vi "VisBx Anzeige PNS.vi"() -> ()   [LabVIEW 2020, in "PNS.lvlib" / "PNS Anlagenuebersicht.lvlib"]
uses:
  PNS Anlagenuebersicht.lvlib
  Visualisierungs Elemente/Zahlen-Ausgabefeld.ctl
  Aktionen FGV Loopkennung.ctl
  Aktionen FGV Grenzwerte.ctl
  Seiten/System Einstellungen V2/Aktioen FGV System.ctl
  PNS Ausgabefelder einfaerben Aktionen.ctl
  <vilib>/Utility/miscctls.llb/LVPointTypeDef.ctl
  Stoerungen/FGV Stoerung aufnehmen Aktion.ctl
  Aktionen FGV Istwerte.ctl
  <vilib>/picture/picture.llb/Draw True-Color Pixmap.vi
  PNS.lvlib
  Allgemein/allgemeine Sub-VIs.lvlib
  Seiten/Anlagenuebersicht/VisBx Anzeige/TDMS laden/TDMS laden.lvlib
  Seiten/Anlagenuebersicht/VisBx Anzeige/VisBx Anzeige.lvlib
  Stoerungen/Stoerungen.lvlib
  Seiten/System Einstellungen V2/System Einstellungen V2.lvlib
  Seiten/Anlagenuebersicht/VisBx Anzeige/Anlagenuebersicht.lvlib
panel:
  out "maxLoop":i32=10
  out "PNS Inaktiv":string
  out "Komm":string
  out "Druckluft":string
  in  "Fehler":string="Die Umgebungsvariable besitzt\nnicht den selben Datentyp wie\ndie TDMS-Datei."
  out "°C":T1
  out "°C":T1
  out "°C":T1
  out "°C":T1
  out "°C":T1
  out "°C":T1
  out "°C":T1
  out "°C":T1
  out "Bild":picture
  # "Anlagenübersicht PNS"
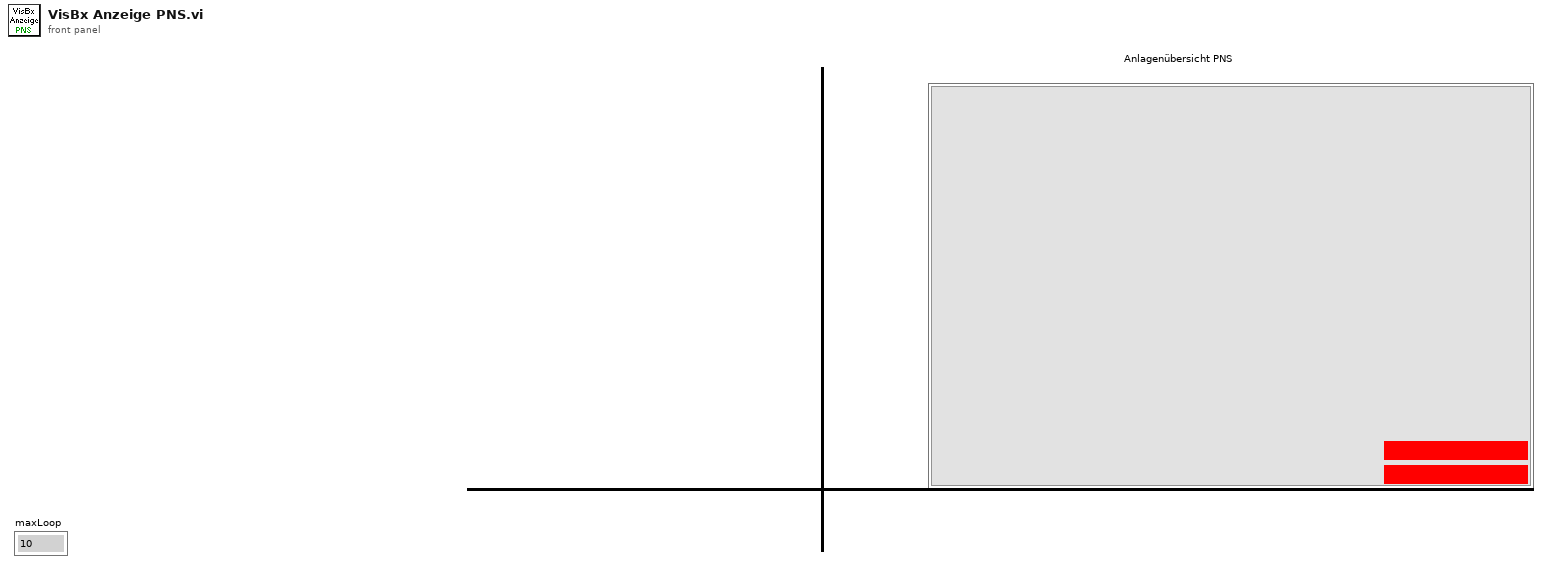
[diagram p1: front panel]
types:
  T1 = typedef "Zahlen-Ausgabefeld.ctl" = sgl
  T2 = typedef "PNS.lvlib/Aktionen FGV Loopkennung.ctl" = enum16{"lesen", "schreiben"}
  T3 = typedef "PNS.lvlib/PNS Anlagenuebersicht.lvlib/PNS Ausgabefelder einfaerben Aktionen.ctl" = enum16{"lesen", "prüfen", "initialisieren"}
  T4 = typedef "System Einstellungen V2.lvlib/Aktioen FGV System.ctl" = enum16{"lesen", "laden", "speichern", "Optionen schreiben", "Zeitstempel", "Reset BMP", "Reset SQP", "Wartung", "Werkseinstellung"}
  T5 = typedef "PNS.lvlib/Aktionen FGV Grenzwerte.ctl" = enum16{"lesen", "Grenzw. schreiben", "Anweisungscode", "IP-Adresse", "laden", "speichern", "Anweisungscode vorgeben"}
  T6 = typedef "LVPointTypeDef.ctl" = cluster{"Horizontal":i16, "Vertical":i16}
  T7 = typedef "PNS.lvlib/PNS Geraetekennung.ctl" = cluster{"Loops":string[], "Gerätetype":string, "Loopkennung":u16[], "Seriennummer":string, "Geraetekennung":u16, "SoftWare Version":string, "LP Kennung":u16}
  T8 = typedef "System Einstellungen V2.lvlib/Optionen.ctl" = cluster{"Störmeldep.":bool, "Betriebszustände":bool, "LN2 Befüllung":bool, "Klimaanlage ?":bool, "AK in ppm":bool, "log Cal-Gas":bool, "log 0-Gas":bool, "log CG zu PNS":bool, "Reserve":bool, "Durchflusssensor 0-5V":bool, "PNS?":bool, "Container":bool, "Mit N2 spülen":bool, "Span Gas Auswahl":T9, "VFS 1":bool, "VFS 2":bool, "VFS 3":bool, "VFS 4":bool, "TRE08":bool, "Leakcheck vor Kal":bool, "Amium 10-Fach":bool, "Verticale Scrollbar aktiv":bool, "Loggingtakt":bool, "SP laden speichern":u16}
  T9 = typedef "Funktionstasten.lvlib/Spaneingang.ctl" = u16
  T10 = typedef "Steuerung PNS.lvclass/Anlegengrenzwerte PNS.ctl" = cluster{"Filter:":T11, "Ventilplatte:":T11, "Heizleitung 1:":T11, "Heizleitung 2:":T11, "Heizleitung 3:":T11, "Heizleitung 4:":T11, "Heizleitung 5:":T11, "Heizleitung 6:":T11}
  T11 = typedef "Steuerung PNS.lvclass/Anlagengrenzwerte Parameteranzeige.ctl" = cluster{"Sollwert":T12, "Warn-Min":T12, "Warn-Max":T12, "Abschalt-Min":T12, "Abschalt-Max":T12, "Regler":u16, "AnlagenParameter":string}
  T12 = typedef "Zahlen-Eingabefeld.ctl" = sgl
  T13 = typedef "VisParam-Typdef.lvlib/VisSchritt.ctl" = cluster{"Schritt-Typ":T14, "Schritt-Daten":variant}
  T14 = typedef "VisParam-Typdef.lvlib/VisSchritt-Typ.ctl" = enum16{"leer", "Punkt", "Linie", "Linienzug", "Fixtext", "Textrechteck", "Ziffernanzeige", "Rechteck", "Rechteck rund", "Ellipse", "Bogen", "Kreis", "Pixmap"}
  T15 = typedef "Anlagenuebersicht.lvlib/VisBx Anzeige.lvlib/TDMS laden.lvlib/TDMS-Eigenschaften.ctl" = cluster{"Größe":T16, "URL":string, "Raster":i16, "Hintergrund":u32}
  T16 = typedef "LVBoundsTypeDef.ctl" = cluster{"Width":u32, "Height":u32}
  T17 = typedef "PNS.lvlib/Aktionen FGV Istwerte.ctl" = enum16{"lesen", "initialisieren", "schreiben", "Störungen"}
  T18 = typedef "Stoerungen.lvlib/FGV Stoerung aufnehmen Aktion.ctl" = enum16{"Initialisieren", "Schreiben", "Lesen", "Quittieren", "quit. löschen"}
  T19 = typedef "Steuerung PNS.lvclass/Regler.ctl" = cluster{"Istwert":i16, "Sollwert":i16, "Alarm MIN":i16, "Alarm MAX":i16, "Regler sperren":i16, "Analog Ausgang":i16}[]
  T20 = cluster{"Istwert":i16, "Sollwert":i16, "Alarm MIN":i16, "Alarm MAX":i16, "Regler sperren":i16, "Analog Ausgang":i16}
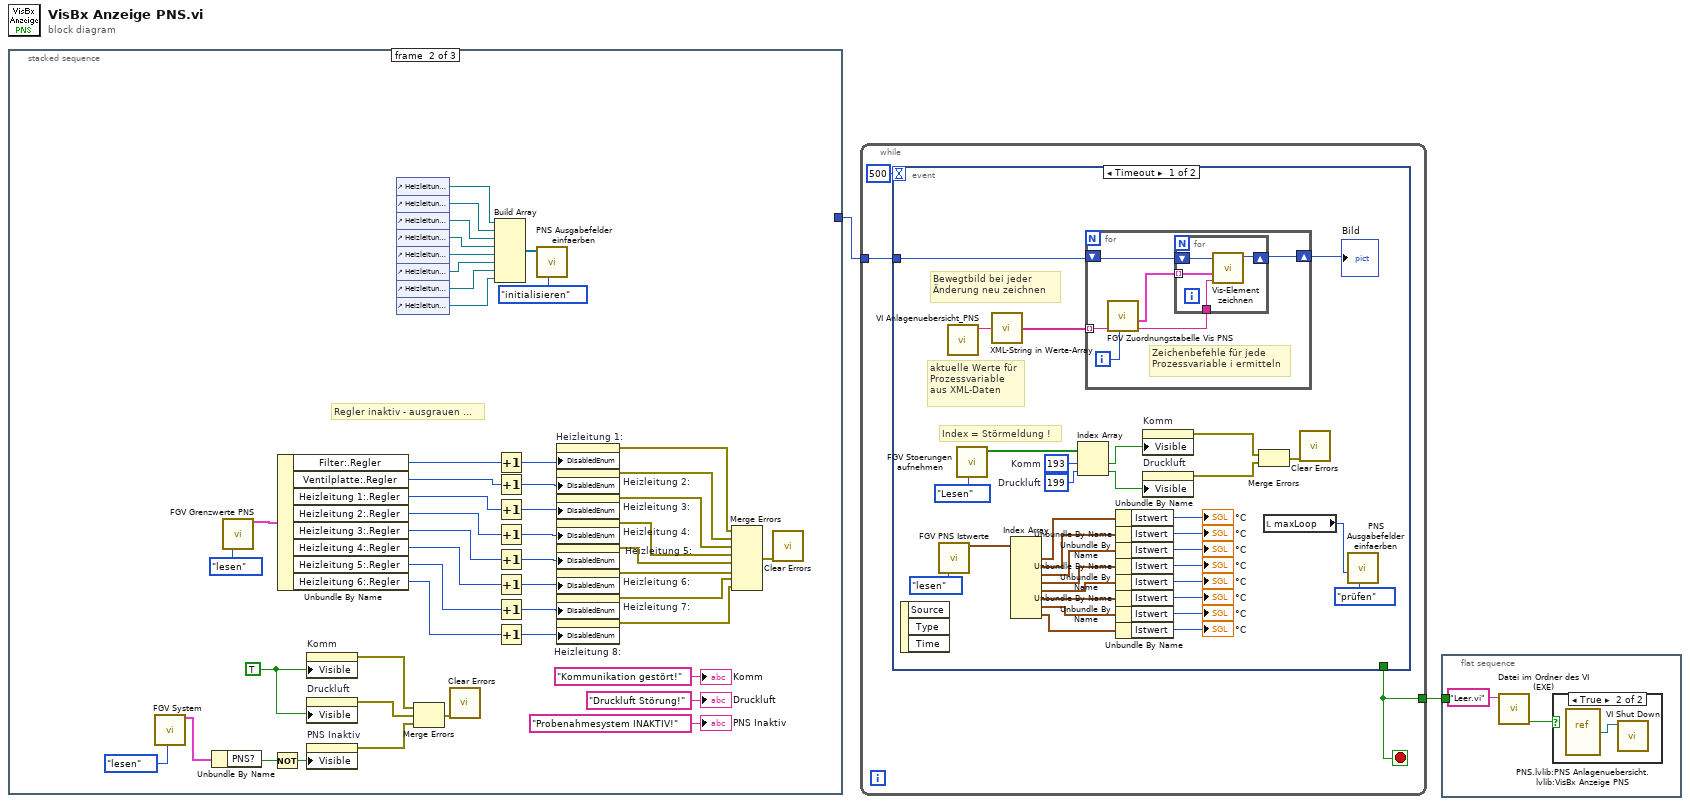
[diagram p0: block diagram]
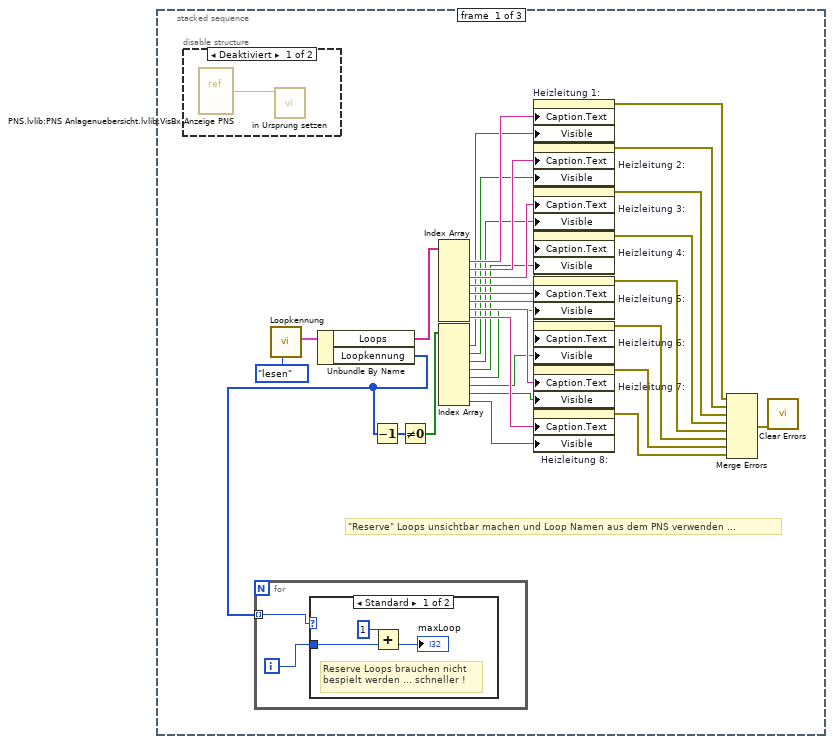
[diagram p3: hidden frame]
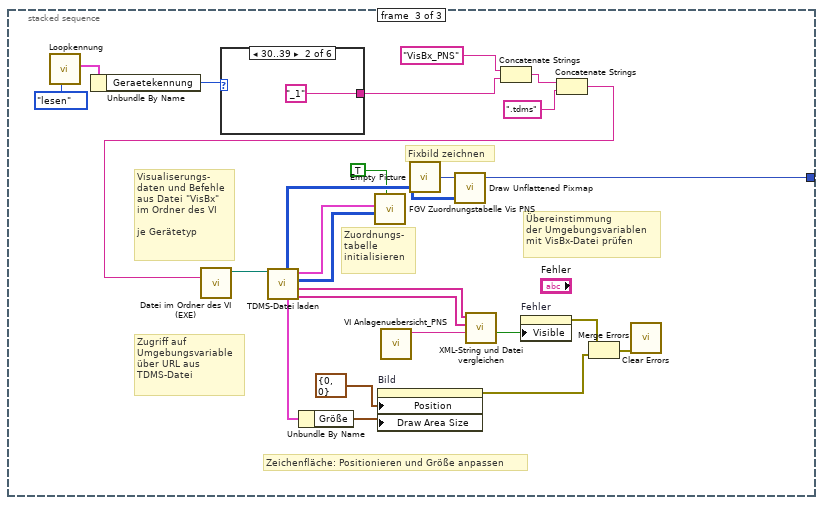
[diagram p6: hidden frame]
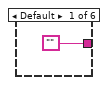
[diagram p7: hidden frame]
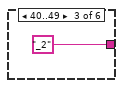
[diagram p8: hidden frame]
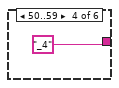
[diagram p9: hidden frame]
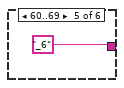
[diagram p10: hidden frame]
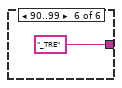
[diagram p11: hidden frame]
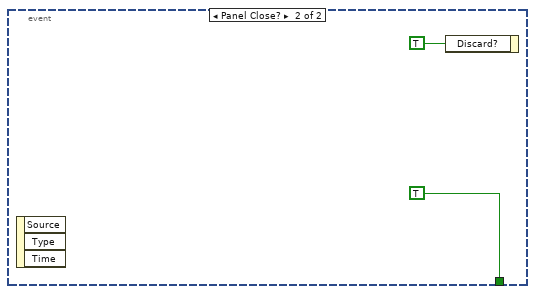
[diagram p12: hidden frame]
diagram:
  n1 = stacked-sequence {
    tunnel: [_ _ w105] -> w2
    frame #0 {
      # "\"Reserve\" Loops unsichtbar machen und Loop Namen aus dem PNS verwenden ..."
      n2 = disable-structure shown="Deaktiviert" {
        frame Disabled {
          n3 = vi-ref "PNS.lvlib:PNS Anlagenuebersicht.lvlib:VisBx Anzeige PNS.vi"() -> (w39:refnum<vi>)
          n4 = call "in Ursprung setzen.vi"("VI Referenz"=w39) -> ()  [unwired: 11 in]
        }
        frame Enabled {
        }
      }
      n5 = call "Loopkennung.vi"("Aktion"=Aktionen_FGV_Loopkennung."lesen") -> ("LoopGeraetekennung"=w32:T7)  [unwired: 9 in, 1 out]
      n6 = Unbundle By Name(w32) -> ("Loops"=w31:string[], "Loopkennung"=w3:u16[])
      n7 = for {
        tunnel: w3 -> [w35] mode=indexing
        i -> [w34]
        n8 = case shown="Standard" w35 {
          tunnel: w34 -> [w38 _]
          frame Default {
            # "Reserve Loops brauchen nicht\nbespielt werden ... schneller !"
            n9 = Add(x=1, y=w38) -> (x+y=→"maxLoop":i32)
          }
          frame 1 {
            # "Reserve Loop,\nmaxLoop nicht mehr \nhoch zählen ..."
          }
        }
      }
      n10 = Decrement(x=w3) -> (x-1=w13:u16[])
      n11 = Not Equal To 0?(x=w13) -> (x != 0?=w12:bool[])
      n12 = Index Array(array=w31) -> (element #1=w23:string, element #2=w24:string, element #3=w25:string, element #4=w26:string, element #5=w30:string, element #6=w29:string, element #7=w28:string, element #8=w27:string)  [unwired: 8 in]
      n13 = Index Array(array=w12) -> (element #1=w11:bool, element #2=w10:bool, element #3=w9:bool, element #4=w8:bool, element #5=w7:bool, element #6=w6:bool, element #7=w5:bool, element #8=w4:bool)  [unwired: 8 in]
      n14 = property on="Heizleitung 1:" class="DigWert (strikt)"("Caption.Text"=w23, "Visible"=w11) -> (error out=w21:errorcluster)  [unwired: 2 in, 1 out]
      n15 = property on="Heizleitung 2:" class="DigWert (strikt)"("Caption.Text"=w24, "Visible"=w10) -> (error out=w20:errorcluster)  [unwired: 2 in, 1 out]
      n16 = property on="Heizleitung 3:" class="DigWert (strikt)"("Caption.Text"=w25, "Visible"=w9) -> (error out=w19:errorcluster)  [unwired: 2 in, 1 out]
      n17 = property on="Heizleitung 4:" class="DigWert (strikt)"("Caption.Text"=w26, "Visible"=w8) -> (error out=w18:errorcluster)  [unwired: 2 in, 1 out]
      n18 = property on="Heizleitung 5:" class="DigWert (strikt)"("Caption.Text"=w30, "Visible"=w7) -> (error out=w17:errorcluster)  [unwired: 2 in, 1 out]
      n19 = property on="Heizleitung 6:" class="DigWert (strikt)"("Caption.Text"=w29, "Visible"=w6) -> (error out=w16:errorcluster)  [unwired: 2 in, 1 out]
      n20 = property on="Heizleitung 7:" class="DigWert (strikt)"("Caption.Text"=w28, "Visible"=w5) -> (error out=w15:errorcluster)  [unwired: 2 in, 1 out]
      n21 = property on="Heizleitung 8:" class="DigWert (strikt)"("Caption.Text"=w27, "Visible"=w4) -> (error out=w14:errorcluster)  [unwired: 2 in, 1 out]
      n22 = Merge Errors(w21, w20, w19, w18, w17, w16, w15, w14) -> (w22:errorcluster)
      n23 = call <vilib>:"Clear Errors.vi"("error in (no error)"=w22) -> ()  [unwired: 5 in, 2 out]
    }
    frame #1 {
      w54 = TRUE
      # "Regler inaktiv - ausgrauen ..."
      n24 = call "FGV System.vi"("Aktionen"=Aktioen_FGV_System."lesen") -> ("Optionen"=w53:T8)  [unwired: 12 in, 6 out]
      n25 = Unbundle By Name(w53) -> ("PNS?"=w51:bool)
      n26 = call "FGV Grenzwerte PNS.vi"("Aktionen FGV Grenzwerte"=Aktionen_FGV_Grenzwerte."lesen") -> ("Grenzwerte PNS 2"=w79:T10)  [unwired: 12 in, 2 out]
      n27 = Not(x=w51) -> (.not. x?=w68:bool)
      n28 = Unbundle By Name(w79) -> ("Filter:.Regler"=w78:u16, "Ventilplatte:.Regler"=w77:u16, "Heizleitung 1:.Regler"=w76:u16, "Heizleitung 2:.Regler"=w75:u16, "Heizleitung 3:.Regler"=w74:u16, "Heizleitung 4:.Regler"=w73:u16, "Heizleitung 5:.Regler"=w72:u16, "Heizleitung 6:.Regler"=w81:u16)
      n29 = property on="Komm" class="Str"("Visible"=w54) -> (error out=w66:errorcluster)  [unwired: 2 in, 1 out]
      n30 = property on="Druckluft" class="Str"("Visible"=w54) -> (error out=w65:errorcluster)  [unwired: 2 in, 1 out]
      n31 = property on="PNS Inaktiv" class="Str"("Visible"=w68) -> (error out=w64:errorcluster)  [unwired: 2 in, 1 out]
      n32 = control-ref of="Heizleitung 1:"() -> (w46:refnum<vi>)
      n33 = control-ref of="Heizleitung 2:"() -> (w48:refnum<vi>)
      n34 = control-ref of="Heizleitung 3:"() -> (w47:refnum<vi>)
      n35 = control-ref of="Heizleitung 4:"() -> (w44:refnum<vi>)
      n36 = control-ref of="Heizleitung 5:"() -> (w43:refnum<vi>)
      n37 = control-ref of="Heizleitung 6:"() -> (w42:refnum<vi>)
      n38 = control-ref of="Heizleitung 7:"() -> (w41:refnum<vi>)
      n39 = control-ref of="Heizleitung 8:"() -> (w40:refnum<vi>)
      n40 = Merge Errors(w66, w65, w64) -> (w67:errorcluster)
      n41 = call <vilib>:"Clear Errors.vi"("error in (no error)"=w67) -> ()  [unwired: 5 in, 2 out]
      n42 = Build Array(w46, w48, w47, w44, w43, w42, w41, w40) -> (w45:refnum<vi>[])
      n43 = Increment(x=w78) -> (x+1=w50:u16)
      n44 = Increment(x=w77) -> (x+1=w82:u16)
      n45 = Increment(x=w76) -> (x+1=w83:u16)
      n46 = Increment(x=w75) -> (x+1=w84:u16)
      n47 = Increment(x=w74) -> (x+1=w85:u16)
      n48 = Increment(x=w73) -> (x+1=w86:u16)
      n49 = Increment(x=w72) -> (x+1=w87:u16)
      n50 = Increment(x=w81) -> (x+1=w88:u16)
      n51 = call "PNS Ausgabefelder einfaerben.vi"("Aktionen"=PNS_Ausgabefelder_einfaerben_Aktionen."initialisieren", "Angehängtes Array"=w45) -> ()  [unwired: 10 in]
      n52 = property on="Heizleitung 1:" class="DigWert (strikt)"("DisabledEnum"=w50) -> (error out=w62:errorcluster)  [unwired: 2 in, 1 out]
      n53 = property on="Heizleitung 2:" class="DigWert (strikt)"("DisabledEnum"=w82) -> (error out=w61:errorcluster)  [unwired: 2 in, 1 out]
      n54 = property on="Heizleitung 3:" class="DigWert (strikt)"("DisabledEnum"=w83) -> (error out=w60:errorcluster)  [unwired: 2 in, 1 out]
      n55 = property on="Heizleitung 4:" class="DigWert (strikt)"("DisabledEnum"=w84) -> (error out=w59:errorcluster)  [unwired: 2 in, 1 out]
      n56 = property on="Heizleitung 5:" class="DigWert (strikt)"("DisabledEnum"=w85) -> (error out=w58:errorcluster)  [unwired: 2 in, 1 out]
      n57 = property on="Heizleitung 6:" class="DigWert (strikt)"("DisabledEnum"=w86) -> (error out=w57:errorcluster)  [unwired: 2 in, 1 out]
      n58 = property on="Heizleitung 7:" class="DigWert (strikt)"("DisabledEnum"=w87) -> (error out=w56:errorcluster)  [unwired: 2 in, 1 out]
      n59 = property on="Heizleitung 8:" class="DigWert (strikt)"("DisabledEnum"=w88) -> (error out=w55:errorcluster)  [unwired: 2 in, 1 out]
      n60 = Merge Errors(w62, w61, w60, w59, w58, w57, w56, w55) -> (w63:errorcluster)
      n61 = call <vilib>:"Clear Errors.vi"("error in (no error)"=w63) -> ()  [unwired: 5 in, 2 out]
      "Druckluft" <- "Druckluft Störung!" ("Druckluft")
      "Komm" <- "Kommunikation gestört!" ("Komm")
      "PNS Inaktiv" <- "Probenahmesystem INAKTIV!" ("Druckluft")
    }
    frame #2 {
      # "Übereinstimmung\nder Umgebungsvariablen\nmit VisBx-Datei prüfen"
      # "Zeichenfläche: Positionieren und Größe anpassen"
      # "Zuordnungs-\ntabelle\ninitialisieren"
      # "Fixbild zeichnen"
      # "Zugriff auf\nUmgebungsvariable\nüber URL aus\nTDMS-Datei"
      # "Visualiserungs-\ndaten und Befehle\naus Datei \"VisBx\"\nim Ordner des VI\n\nje Gerätetyp"
      n62 = call "Loopkennung.vi"("Aktion"=Aktionen_FGV_Loopkennung."lesen") -> ("LoopGeraetekennung"=w97:T7)  [unwired: 9 in, 1 out]
      n63 = Unbundle By Name(w97) -> ("Geraetekennung"=w96:u16)
      n64 = case shown="30..39" w96 {
        tunnel: ["" "_1" "_2" "_4" "_6" "_TRE"] -> w94
        frame Default {
        }
        frame 30..39 {
        }
        frame 40..49 {
        }
        frame 50..59 {
        }
        frame 60..69 {
        }
        frame 90..99 {
        }
      }
      n65 = call "VI Anlagenuebersicht_PNS.vi"() -> ("XML-String"=w107:string)  [unwired: 11 in]
      n66 = call "Empty Picture"() -> ("empty picture"=w112:picture)
      n67 = Concatenate Strings("VisBx_PNS" ("Dateiname"), w94) -> (w93:string)
      n68 = Concatenate Strings(w93, ".tdms" ("Dateiname")) -> (w92:string)
      n69 = call "Datei im Ordner des VI (EXE).vi"("Dateiname"=w92) -> ("Dateipfad im Ordner des Haupt-VIs"=w113:path)  [unwired: 8 in, 2 out]
      n70 = call "TDMS-Datei laden.vi"("Dateipfad"=w113) -> ("Datentypen"=w108:string[], "Namen"=w109:string[], "Zuordnungstabelle"=w110:i16[][], "Programm"=w111:T13[], "Eigenschaften"=w106:T15, "Fixbild (Pixmap)"=w98:u32[][])  [unwired: 4 in, 1 out]
      n71 = Unbundle By Name(w106) -> ("Größe"=w101:T16)
      n72 = call "FGV Zuordnungstabelle Vis PNS.vi"("Initialisieren"=TRUE, "Zuordnungtabelle (init)"=w110, "Programm (init)"=w111) -> ()  [unwired: 6 in, 3 out]
      n73 = property on="Bild" class="Bild"("Position"=T6 {"Horizontal"=0, "Vertical"=0} ("Ursprung"), "Draw Area Size"=w101) -> (error out=w99:errorcluster)  [unwired: 2 in, 1 out]
      n74 = call-poly <vilib>:"Draw Unflattened Pixmap.vi"("picture"=w112, "data (RGB format)"=w98) -> ("new picture"=w105:picture)  [unwired: 7 in]
      n75 = call "XML-String und Datei vergleichen.vi"("XML-String"=w107, "Datentypen aus Datei"=w108, "Namen aus Datei"=w109) -> ("nicht gleich"=w102:bool)  [unwired: 6 in, 2 out]
      n76 = property on="Fehler" class="Str"("Visible"=w102) -> (error out=w103:errorcluster)  [unwired: 2 in, 1 out]
      n77 = Merge Errors(w103, w99) -> (w104:errorcluster)
      n78 = call <vilib>:"Clear Errors.vi"("error in (no error)"=w104) -> ()  [unwired: 5 in, 2 out]
    }
  }
  n79 = while {
    tunnel: w2 -> [w121]
    tunnel: [w120] -> w1
    stop <- w120 stop-if-true
    n80 = event shown="[0] Timeout" {
      selector: _ -> [_ _]
      dyn-events: _ -> [_ _]
      timeout: 500 -> [_ _]
      tunnel: w121 -> [w135 _]
      tunnel: [_ TRUE] -> w120
      event Timeout {
        w131 = 199  # Druckluft
        w132 = 193  # Komm
        # "Index = Störmeldung !"
        # "Bewegtbild bei jeder\nÄnderung neu zeichnen"
        # "aktuelle Werte für\nProzessvariable\naus XML-Daten"
        n81 = event-data() -> ()  [unwired: 1 in, 3 out]
        n82 = call "FGV PNS Istwerte.vi"("Aktionen"=Aktionen_FGV_Istwerte."lesen") -> ("Regler"=w155:T19)  [unwired: 11 in, 3 out]
        n83 = call "VI Anlagenuebersicht_PNS.vi"() -> ("XML-String"=w137:string)  [unwired: 11 in]
        n84 = call "FGV Stoerungen aufnehmen.vi"("FGV Störung aufnehmen Aktion"=FGV_Stoerung_aufnehmen_Aktion."Lesen") -> ("aktive Störungen"=w130:bool[])  [unwired: 7 in, 3 out]
        n85 = call "XML-String in Werte-Array.vi"("XML-String"=w137) -> ("Werte"=w136:string[])
        n86 = Index Array(array=w155) -> (element #1=w154:T20, element #2=w153:T20, element #3=w152:T20, element #4=w151:T20, element #5=w150:T20, element #6=w149:T20, element #7=w148:T20, element #8=w139:T20)  [unwired: 8 in]
        n87 = Index Array(array=w130, index #1=w132, index #2=w131) -> (element #1=w129:bool, element #2=w128:bool)
        n88 = for {
          tunnel: w136 -> [w161] mode=indexing
          shift-right: [w158] -> w134
          shift-left: w135 -> [w159]
          i -> [w160]
          # "Zeichenbefehle für jede\nProzessvariable i ermitteln"
          n89 = call "FGV Zuordnungstabelle Vis PNS.vi"("Prozessvariable Nr. N"=w160, "Wert (N)"=w161) -> ("Wert für zeichnen"=w156:string, "Zeichenbefehle"=w157:T13[])  [unwired: 7 in, 1 out]
          n90 = for {
            shift-right: [w164] -> w158
            shift-left: w159 -> [w165]
            tunnel: w157 -> [w163] mode=indexing
            tunnel: w156 -> [w162]
            n91 = call "Vis-Element zeichnen.vi"("Wert-String"=w162, "Schritt"=w163, "Bild alt"=w165) -> ("Bild neu"=w164:picture)  [unwired: 8 in]
          }
        }
        "Bild" <- w134
        n92 = Unbundle By Name(w154) -> ("Istwert"=→"°C":i16)
        n93 = Unbundle By Name(w153) -> ("Istwert"=→"°C":i16)
        n94 = Unbundle By Name(w152) -> ("Istwert"=→"°C":i16)
        n95 = Unbundle By Name(w151) -> ("Istwert"=→"°C":i16)
        n96 = Unbundle By Name(w150) -> ("Istwert"=→"°C":i16)
        n97 = Unbundle By Name(w149) -> ("Istwert"=→"°C":i16)
        n98 = Unbundle By Name(w148) -> ("Istwert"=→"°C":i16)
        n99 = Unbundle By Name(w139) -> ("Istwert"=→"°C":i16)
        n100 = property on="Komm" class="Str"("Visible"=w129) -> (error out=w126:errorcluster)  [unwired: 2 in, 1 out]
        n101 = property on="Druckluft" class="Str"("Visible"=w128) -> (error out=w125:errorcluster)  [unwired: 2 in, 1 out]
        n102 = Merge Errors(w126, w125) -> (w127:errorcluster)
        n103 = local read "maxLoop"() -> (w124:i32)
        n104 = call <vilib>:"Clear Errors.vi"("error in (no error)"=w127) -> ()  [unwired: 5 in, 2 out]
        n105 = call "PNS Ausgabefelder einfaerben.vi"("Aktionen"=PNS_Ausgabefelder_einfaerben_Aktionen."prüfen", "maxLoop"=w124) -> ()  [unwired: 10 in]
      }
      event Panel Close? {
        n106 = event-data() -> ()  [unwired: 1 in, 3 out]
        n107 = event-data("Discard?"=TRUE) -> ()  [unwired: 1 in, 1 out]
      }
    }
  }
  n108 = flat-sequence {
    tunnel: w1 -> [_]
    frame #0 {
      n109 = call "Datei im Ordner des VI (EXE).vi"("Dateiname"="Leer.vi") -> ("EXE"=w168:bool)  [unwired: 8 in, 2 out]
      n110 = case shown="True" w168 {
        frame False {
        }
        frame True {
          n111 = vi-ref "PNS.lvlib:PNS Anlagenuebersicht.lvlib:VisBx Anzeige PNS.vi"() -> (w170:refnum<vi>)
          n112 = call "VI Shut Down.vi"("VI Referenz"=w170) -> ()  [unwired: 11 in]
        }
      }
    }
  }
